vi "WPI_I2CEnumerate.vi"(10 "I2C Bus":T1=enum."Invalid") -> (2 "Discovered Devices":i32[](array[numeric]))   [LabVIEW 2017]
doc: "Enumerates a list of attached I2C devices by address."
uses:
  <vilib>/Rock Robotics/SystemInterfaces/i2clib/i2c_bus.ctl
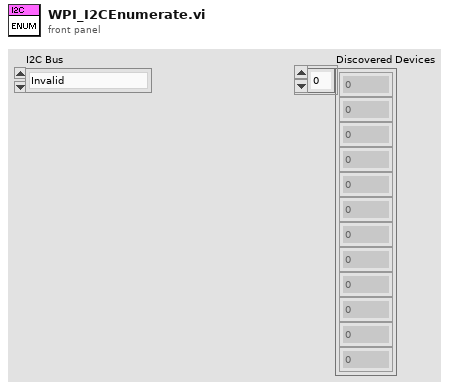
[diagram p1: front panel]
types:
  T1 = typedef "i2c_bus.ctl" = enum16{"I2C On-Board", "I2C MXP", "Invalid"}
  T2 = typedef "WPI_I2CDevRef.ctl" = cluster{"DevStatus":errorcluster, "Device Address":u8, "Handle":i32, "I2C Bus":T1}
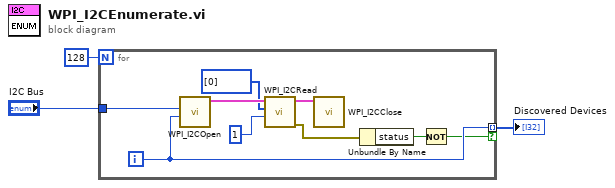
[diagram p0: block diagram]
diagram:
  n1 = for {
    N: 128 -> [_]
    tunnel: [w7] -> w2 mode=indexing if=w5
    tunnel: "I2C Bus" -> [w4]
    i -> [w7]
    n2 = call <vilib>:"WPI_I2COpen.vi"("Device Address"=w7, "I2C Bus"=w4) -> ("I2CDevRef"=w12:T2)  [unwired: 8 in, 1 out]
    n3 = call <vilib>:"WPI_I2CRead.vi"("I2CBytesToRead"=u8 1, "I2CRegister"=u8[] [0], "I2CDevRef"=w12) -> ("error out"=w8:errorcluster, "I2CDevRef"=w11:T2)  [unwired: 6 in, 1 out]
    n4 = call <vilib>:"WPI_I2CClose.vi"("I2CDevRef"=w11) -> ()  [unwired: 10 in, 1 out]
    n5 = Unbundle By Name(w8) -> ("status"=w6:bool)
    n6 = Not(x=w6) -> (.not. x?=w5:bool)
  }
  "Discovered Devices" <- w2
